vi "calculate_c_hat.vi"(8 "Error In":errorcluster, 9 "phi_in":dbl, 10 "phi_c":dbl, 11 "theta_c":dbl) -> (0 "Error Out":errorcluster, 3 "c hat":dbl[](array[numeric]))   [LabVIEW 2019]
doc: "Calculate phi from formula 4 in Wilen(2000). All inputs and outputs are in degrees."
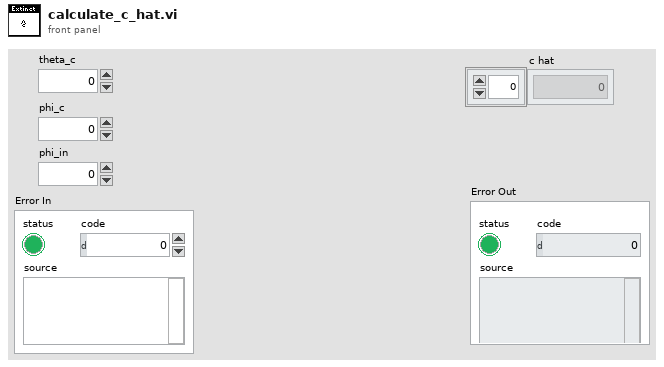
[diagram p1: front panel]
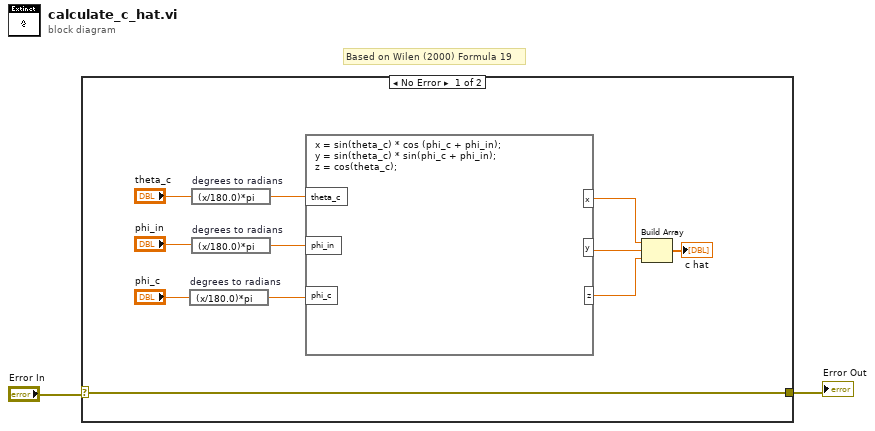
[diagram p0: block diagram]
diagram:
  # "Based on Wilen (2000) Formula 19"
  n1 = case shown="No Error" "Error In" {
    selector: "Error In" -> [w13 w14]
    tunnel: [w13 w14] -> w1
    frame No Error {
      n2 = expression code="(x/180.0)*pi" "degrees to radians"("phi_c") -> (w7:dbl)
      n3 = expression code="(x/180.0)*pi" "degrees to radians"("theta_c") -> (w12:dbl)
      n4 = expression code="(x/180.0)*pi" "degrees to radians"("phi_in") -> (w11:dbl)
      n5 = formula code="x = sin(theta_c) * cos (phi_c + phi_in);\ny = sin(theta_c) * sin(phi_c + phi_in);\nz = cos(theta_c);"("theta_c"=w12, "phi_in"=w11, "phi_c"=w7) -> ("x"=w5:dbl, "y"=w6:dbl, "z"=w4:dbl)
      n6 = Build Array(w5, w6, w4) -> (→"c hat":dbl[])
    }
    frame Error {
    }
  }
  "Error Out" <- w1
